vi "CAN start.vi"(4 "error in (no error)":errorcluster, 7 "CANopen in":refnum<class "CANopen.lvclass">) -> (0 "error out":errorcluster, 3 "CANopen out":refnum<class "CANopen.lvclass">)   [LabVIEW 2026, in "canopen_.lvlib" / "CANopen.lvclass"]
doc: "Starts the internal task that reads and manages the relevant CANopen messages. Furthermore, this will also start the monitoring of heartbeat messages, if the heartbeat table has been set.\n\n\"CAN start\" is not required if you do not intend to handle incoming messages."
uses:
  CANopen.lvclass
  CANopen.lvclass/CANopen.ctl
panel:
  out "Service map":T1(array[cluster])
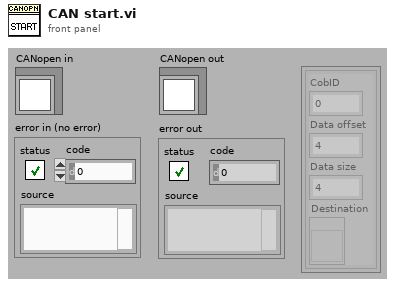
[diagram p1: front panel]
types:
  T1 = cluster{"CobID":u32, "Data offset":u8, "Data size":u8, "Destination":refnum<vi>}[]
  T2 = typedef "Semaphore RefNum" = refnum<k1>
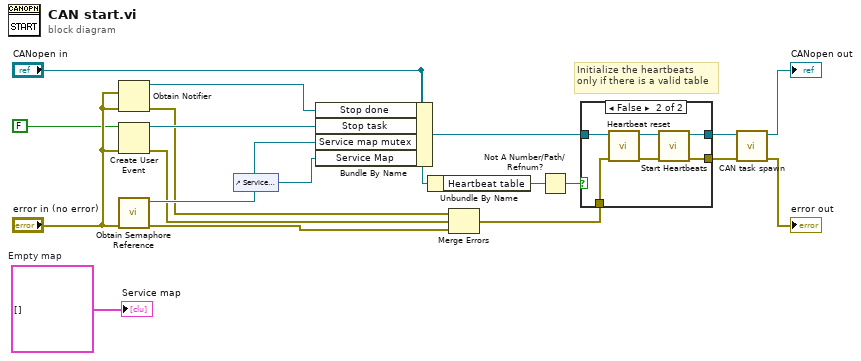
[diagram p0: block diagram]
diagram:
  w16 = T1 []  # Empty map
  # "Initialize the heartbeats\nonly if there is a valid table"
  n1 = Obtain Notifier(notification data type="error in (no error)", error in (no error)="error in (no error)") -> (notifier out=w11:refnum<notifier>, error out=w10:errorcluster)  [unwired: 1 in, 2 out]
  n2 = Create User Event ("Ferma task")(user event datatype=FALSE ("Stop?"), error in="error in (no error)") -> (user event=w19:refnum<user-event>, error out=w13:errorcluster)
  n3 = call <vilib>:"Obtain Semaphore Reference.vi"("error in (no error)"="error in (no error)") -> ("error out"=w14:errorcluster, "semaphore"=w17:T2)  [unwired: 2 in, 3 out]
  n4 = control-ref of="Service map"() -> (w15:refnum<vi>)
  n5 = Bundle By Name(cluster="CANopen in", "Stop done"=w11, "Stop task"=w19, "Service map mutex"=w17, "Service Map"=w15) -> (w7:refnum<class "CANopen.lvclass">)
  n6 = Unbundle By Name("CANopen in") -> ("Heartbeat table"=w1:refnum<vi>)
  n7 = Merge Errors(w10, w13, w14) -> (w9:errorcluster)
  n8 = Not A Number/Path/Refnum?(number/path/refnum=w1) -> (NaN/Path/Refnum?=w2:bool)
  n9 = case shown="False" w2 {
    tunnel: w9 -> [w20 w27]
    tunnel: [w21 w24] -> w8
    tunnel: w7 -> [w21 w23]
    tunnel: [w20 w22] -> w4
    frame True {
    }
    frame False {
      n10 = call "Heartbeat reset.vi"("error in"=w27, "CANopen in"=w23) -> ("error out"=w26:errorcluster, "CANopen out"=w25:refnum<class "CANopen.lvclass">)  [unwired: 1 in, 3 out]
      n11 = call "Start Heartbeats.vi"("error in"=w26, "CANopen in"=w25) -> ("error out"=w22:errorcluster, "CANopen out"=w24:refnum<class "CANopen.lvclass">)  [unwired: 1 in, 3 out]
    }
  }
  n12 = call "CAN task spawn.vi"("error in (no error)"=w4, "CANopen in"=w8) -> ("error out"=→"error out":errorcluster, "CANopen out"=→"CANopen out":refnum<class "CANopen.lvclass">)  [unwired: 4 out]
  "Service map" <- w16
